vi "calc swerve modules.vi"(0 "DRIVER INPUT":T1 {"Jr" format="%.4g"; "theta (rad)" format="%_4f"; "R" format="%.4g"; "Jy" format="%.4g"; "theta (deg)" format="%_4f"; "Jx" format="%.4g"}, 1 "Alliance":T4, 2 "front face":T3, 3 "HDG (deg)":dbl, 5 "error in (no error)":errorcluster, 8 "drive frame":T2, 9 "MAX spin (rev/s)":dbl=0.7000000000000001 format="%#_13g", 10 "Vmax":dbl=0.9999999999999992 format="%#_13g") -> (16 "speed norm":dbl[](array[numeric])=[0.8999999999999999, 0.37570029466522775, 0.37570029466522775, 0.9] format="%.4f", 17 "angle":dbl[](array[numeric])=[111.25110893724829, 150.25858148936936, 29.741418510630655, 68.7488910627517] format="%.4f", 19 "error out":errorcluster)   [LabVIEW 2023]
uses:
  <vilib>/Rock Robotics/WPI/DriverStation/WPI_DriverStationAllianceInfo.ctl
  ctrl defs/ctrl FRONT FACE selector.ctl
  ctrl defs/ctrl DRIVING FRAME selector.ctl
  ctrl defs/ctrl driver input.ctl
  <vilib>/Analysis/coordinate.llb/Angle Units.ctl
  <vilib>/Analysis/coordinate.llb/Angle Range (Degree).ctl
  <vilib>/Analysis/coordinate.llb/Wrap Angle (scalar).vi
  Global odometry.vi
  <vilib>/Analysis/NI_AAL_Angle.lvlib
panel:
  out "PARK":bool
  out "speed":dbl[](array[numeric])=[1.7557882008191608, 0.7329446049083209, 0.7329446049083209, 1.755788200819161] format="%.4f"
  out "straight + rotate":cluster{"X":dbl, "Y":dbl}[](array[cluster])=[{"X"=-0.6363961030678926, "Y"=1.6363961030678928}, {"X"=-0.6363961030678928, "Y"=0.36360389693210726}, {"X"=0.636396103067893, "Y"=0.36360389693210726}, {"X"=0.636396103067893, "Y"=1.6363961030678928}] {"X" format="%.4f"; "Y" format="%.4g"}
  out "theta (deg)":dbl=90.0
  out "rotate":dbl=0.9
  out "rotate XY":cluster{"X":dbl, "Y":dbl}[](array[cluster])=[{"X"=-0.6363961030678927, "Y"=0.6363961030678928}, {"X"=-0.636396103067893, "Y"=-0.6363961030678927}, {"X"=0.6363961030678928, "Y"=-0.6363961030678927}, {"X"=0.6363961030678928, "Y"=0.6363961030678927}] {"X" format="%.4g"; "Y" format="%.4g"}
  out "straight XY":cluster{"X":dbl, "Y":dbl}[](array[cluster])=[{"X"=6.123233995736766e-17, "Y"=1.0}, {"X"=6.123233995736766e-17, "Y"=1.0}, {"X"=6.123233995736766e-17, "Y"=1.0}, {"X"=6.123233995736766e-17, "Y"=1.0}] {"X" format="%.4f"; "Y" format="%.4g"}
  out "R CG to mod":dbl[](array[numeric])=[17.273204450824984, 17.273204450824984, 17.273204450824984, 17.273204450824984]
  # "assumes steering position 0 = +X while drive rotates forward"
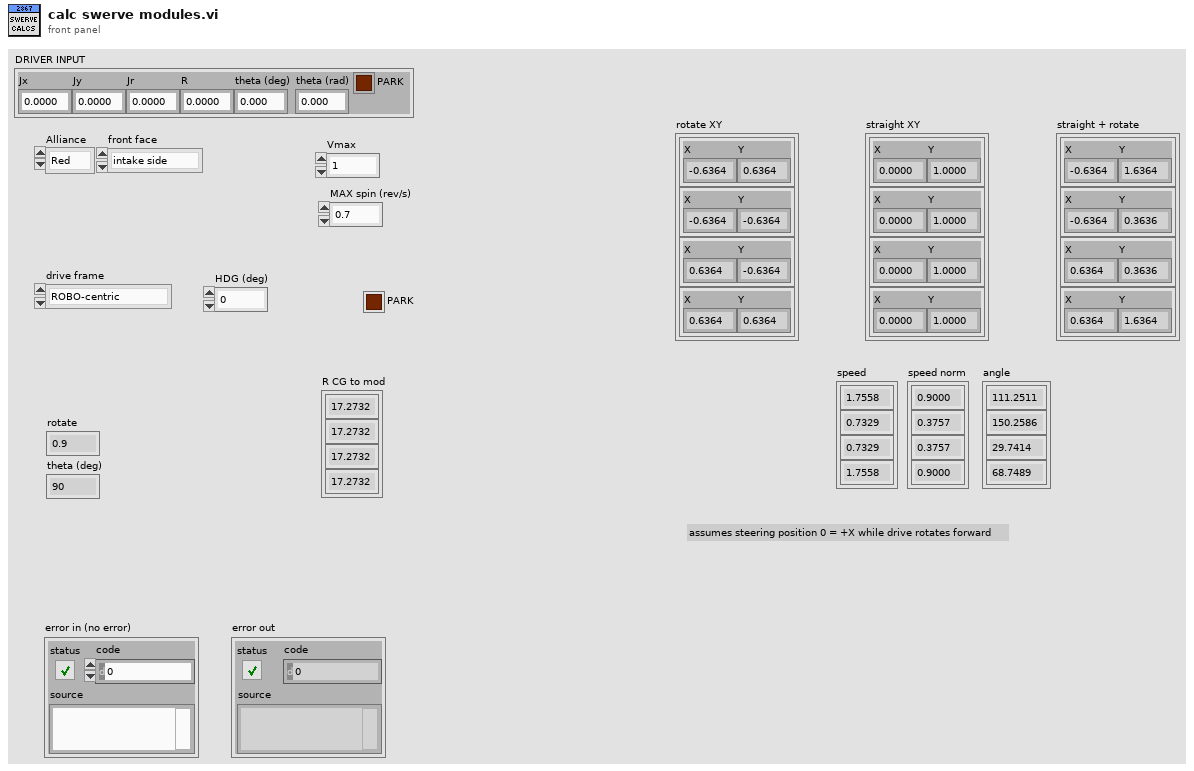
[diagram p1: front panel]
types:
  T1 = typedef "ctrl driver input.ctl" = cluster{"Jx":dbl, "Jy":dbl, "Jr ":dbl, "R":dbl, "theta (deg)":dbl, "theta (rad)":dbl, "PARK":bool}
  T2 = typedef "ctrl DRIVING FRAME selector.ctl" = enum16{"ROBO-centric", "FLD-centric"}
  T3 = typedef "ctrl FRONT FACE selector.ctl" = enum16{"intake side", "shooter side"}
  T4 = typedef "WPI_DriverStationAllianceInfo.ctl" = enum16{"Red", "Blue", "Invalid"}
  T5 = typedef "NI_AAL_Angle.lvlib/Angle Units.ctl" = i32
  T6 = typedef "NI_AAL_Angle.lvlib/Angle Range (Degree).ctl" = u16
  T7 = typedef "ctrl PARKING constants.ctl" = cluster{"angle (deg)":dbl, "%VBus":dbl}
  T8 = typedef "ctrl swerve module.ctl" = cluster{"descr":string, "V":dbl, "POS":dbl, "target":dbl, "ABS":dbl, "from pivot to module":cluster{"R":dbl, "theta (deg)":dbl, "theta spin (deg)":dbl, "theta park (deg)":dbl}, "coord wrt geom CTR":cluster{"X":dbl, "Y":dbl}, "corner wt (lbm)":dbl}
  T9 = cluster{"R":dbl, "theta (deg)":dbl, "theta spin (deg)":dbl, "theta park (deg)":dbl}
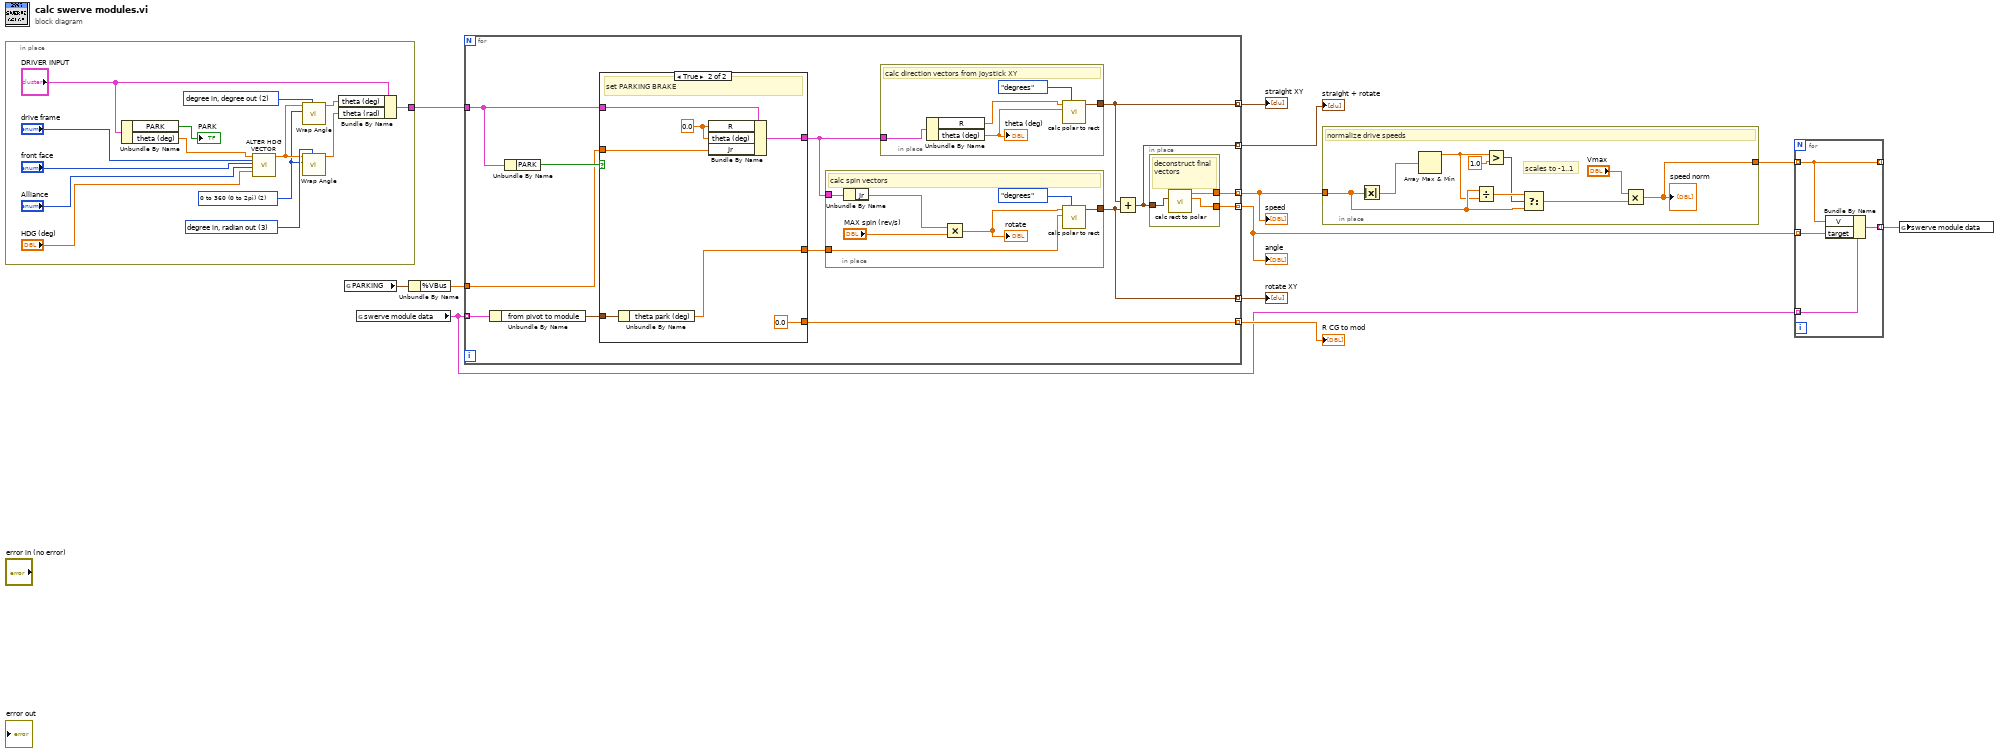
[diagram p0: block diagram]
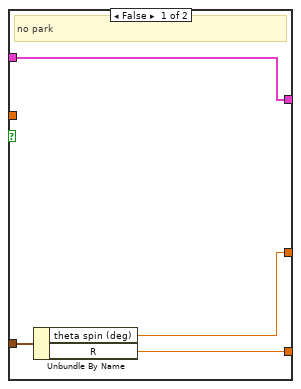
[diagram p2: hidden frame]
diagram:
  n1 = in-place {
    in-place-border: [w26] -> w3
    w14 = T5 2 items=["radian in, radian out", "radian in, degree out", "degree in, degree out", "degree in, radian out"] ("angle units")
    w15 = T6 2 items=["none", "-180 to 180 (-pi to pi)", "0 to 360 (0 to 2pi)"] ("angle range")
    w24 = T5 3 items=["radian in, radian out", "radian in, degree out", "degree in, degree out", "degree in, radian out"] ("angle units")
    n2 = Unbundle By Name("DRIVER INPUT") -> ("PARK"=→"PARK":bool, "theta (deg)"=w22:dbl)
    n3 = call "ALTER HDG VECTOR.vi"("Joystick angle (deg CCW)"=w22, "drive frame"="drive frame", "front face"="front face", "Alliance"="Alliance", "ROBOT compass reading (deg CW)"="HDG (deg)") -> ("Joystick (deg)"=w23:dbl)  [unwired: 14 in]
    n4 = call-poly <vilib>:"Wrap Angle.vi"("angle units"=w14, "angle range"=w15, "angle in"=w23) -> ("angle out"=w16:dbl)  [unwired: 7 in, 1 out]
    n5 = call-poly <vilib>:"Wrap Angle.vi"("angle units"=w24, "angle range"=w15, "angle in"=w23) -> ("angle out"=w25:dbl)  [unwired: 7 in, 1 out]
    n6 = Bundle By Name(cluster="DRIVER INPUT", "theta (deg)"=w16, "theta (rad)"=w25) -> (w26:T1)
  }
  n7 = global read "Global odometry.vi" "PARKING"() -> (w2:T7)
  n8 = global read "Global odometry.vi" "swerve module data"() -> (w7:T8[])
  n9 = Unbundle By Name(w2) -> ("%VBus"=w1:dbl)
  n10 = for {
    tunnel: [w32] -> w8 mode=indexing
    tunnel: w3 -> [w29]
    tunnel: [w39] -> w12 mode=indexing
    tunnel: [w38] -> w11 mode=indexing
    tunnel: [w35] -> w10 mode=indexing
    tunnel: [w37] -> w9 mode=indexing
    tunnel: [w36] -> w4 mode=indexing
    tunnel: w7 -> [w34] mode=indexing
    tunnel: w1 -> [w27]
    n11 = Unbundle By Name(w34) -> ("from pivot to module"=w33:T9)
    n12 = Unbundle By Name(w29) -> ("PARK"=w28:bool)
    n13 = case shown="True" w28 {
      tunnel: w33 -> [w43 w50]
      tunnel: [w42 0.0 ("R")] -> w32
      tunnel: [w41 w49] -> w31
      tunnel: w29 -> [w40 w47]
      tunnel: [w40 w46] -> w30
      tunnel: w27 -> [_ w44]
      frame False {
        # "no park"
        n14 = Unbundle By Name(w43) -> ("theta spin (deg)"=w41:dbl, "R"=w42:dbl)
      }
      frame True {
        w45 = 0.0 ("R")
        # "set PARKING BRAKE"
        n15 = Unbundle By Name(w50) -> ("theta park (deg)"=w49:dbl)
        n16 = Bundle By Name(cluster=w47, "R"=w45, "theta (deg)"=w45, "Jr"=w44) -> (w46:T1)
      }
    }
    n17 = in-place {
      in-place-border: w31 -> [w56]
      in-place-border: w30 -> [w59]
      in-place-border: [w54] -> w38
      # "calc spin vectors"
      n18 = Unbundle By Name(w59) -> ("Jr"=w60:dbl)
      n19 = Multiply(x=w60, y="MAX spin (rev/s)") -> (x*y=w55:dbl)
      "rotate" <- w55
      n20 = call "calc polar to rect.vi"("units"=enum16{"degrees", "radians"}."degrees", "angle"=w56, "mag"=w55) -> ("XY"=w54:cluster{"X":dbl, "Y":dbl})  [unwired: 8 in]
    }
    n21 = in-place {
      in-place-border: w30 -> [w65]
      in-place-border: [w62] -> w39
      # "calc direction vectors from joystick XY"
      n22 = Unbundle By Name(w65) -> ("R"=w63:dbl, "theta (deg)"=w64:dbl)
      "theta (deg)" <- w64
      n23 = call "calc polar to rect.vi"("units"=enum16{"degrees", "radians"}."degrees", "angle"=w64, "mag"=w63) -> ("XY"=w62:cluster{"X":dbl, "Y":dbl})  [unwired: 8 in]
    }
    n24 = Add(x=w39, y=w38) -> (x+y=w35:cluster{"X":dbl, "Y":dbl})
    n25 = in-place {
      in-place-border: w35 -> [w53]
      in-place-border: [w51] -> w37
      in-place-border: [w52] -> w36
      # "deconstruct final vectors"
      n26 = call "calc rect to polar.vi"("XY"=w53) -> ("angle (deg)"=w52:dbl, "Magnitude"=w51:dbl)  [unwired: 8 in, 1 out]
    }
  }
  "R CG to mod" <- w8
  "straight XY" <- w12
  "rotate XY" <- w11
  "straight + rotate" <- w10
  "angle" <- w4
  "speed" <- w9
  n27 = in-place {
    in-place-border: w9 -> [w73]
    in-place-border: [w66] -> w5
    # "scales to -1..1"
    # "normalize drive speeds"
    n28 = Absolute Value(x=w73) -> (abs(x)=w68:dbl[])
    n29 = Array Max & Min(array=w68) -> (max value=w67:dbl)  [unwired: 3 out]
    n30 = Divide(x=w73, y=w67) -> (x/y=w72:dbl[])
    n31 = Greater?(x=w67, y=1.0) -> (0:w71:bool)
    n32 = Select(t=w72, s=w71, f=w73) -> (s? t:f=w74:dbl[])
    n33 = Multiply(x="Vmax", y=w74) -> (x*y=w66:dbl[])
    "speed norm" <- w66
  }
  n34 = for {
    tunnel: [w77] -> w6 mode=indexing
    tunnel: w7 -> [w78] mode=indexing
    tunnel: [w75] -> _ mode=indexing
    tunnel: w5 -> [w75] mode=indexing
    tunnel: w4 -> [w76] mode=indexing
    n35 = Bundle By Name(cluster=w78, "V"=w75, "target"=w76) -> (w77:T8)
  }
  n36 = global write "Global odometry.vi" "swerve module data"(w6) -> ()
